vi "Send YIELD.vi"(8 "error in (no error)":errorcluster, 9 "Yield request":T1={"Invocation Request ID"=0, "Arguments"=[], "ArgumentsKw"="{}", "Options"="{}"}, 11 "WAMP Client in":refnum<class "WAMP Client.lvclass">) -> (0 "error out":errorcluster, 3 "WAMP Client out":refnum<class "WAMP Client.lvclass">)   [LabVIEW 2020, in "wamplv.lvlib" / "WAMP Client.lvclass"]
uses:
  WAMP Client.lvclass
  TypeDef/YIELD request data.ctl
  TypeDef/WAMP Message Codes.ctl
  WAMP Client.lvclass/WAMP Client.ctl
  <vilib>/JDP Science/JSONtext/JSONtext.lvlib
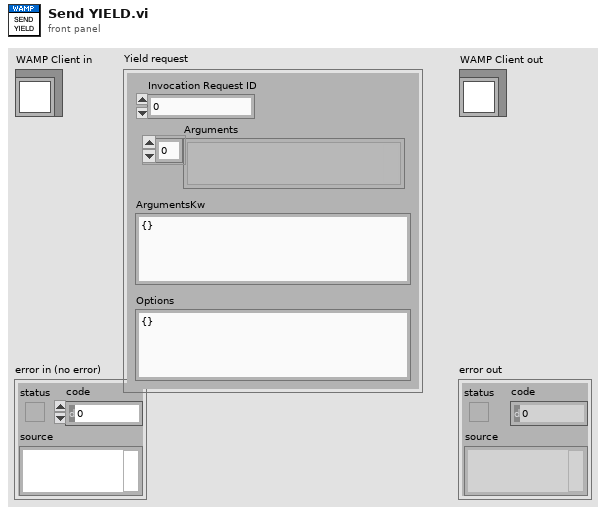
[diagram p1: front panel]
types:
  T1 = typedef "wamplv.lvlib/WAMP Client.lvclass/YIELD request data.ctl" = cluster{"Invocation Request ID":u64, "Arguments":variant[], "ArgumentsKw":string, "Options":string}
  T2 = typedef "wamplv.lvlib/WAMP Client.lvclass/WAMP Message Codes.ctl" = u16
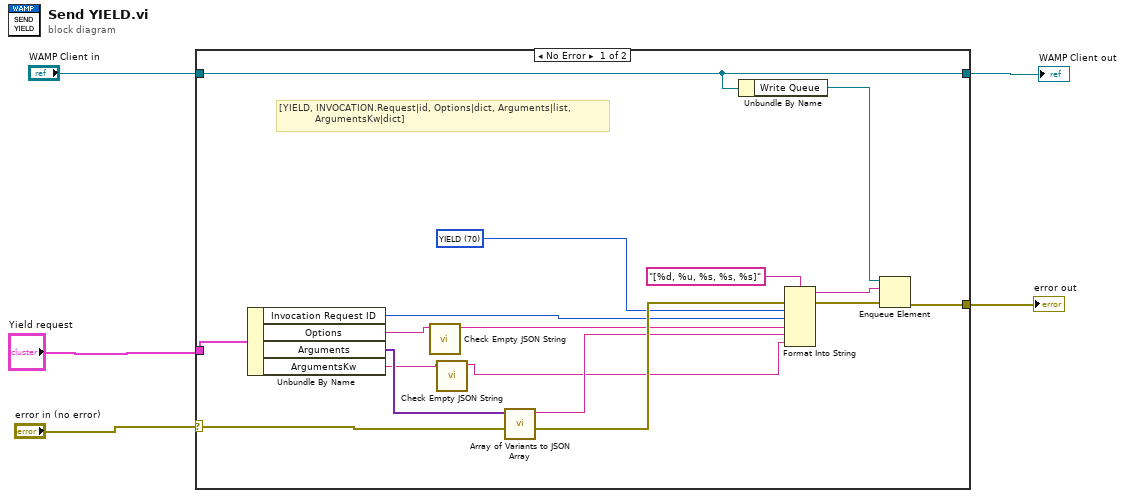
[diagram p0: block diagram]
diagram:
  n1 = case shown="No Error" "error in (no error)" {
    selector: "error in (no error)" -> [w17 w24]
    tunnel: [w22 w24] -> w4
    tunnel: [w15 w23] -> w2
    tunnel: "WAMP Client in" -> [w15 w23]
    tunnel: "Yield request" -> [w13 _]
    frame No Error {
      w14 = T2 70 items=["HELLO"=1, "WELCOME"=2, "ABORT"=3, "GOODBYE"=6, "ERROR"=8, "PUBLISH"=16, "PUBLISHED"=17, "SUBSCRIBE"=32, "SUBSCRIBED"=33, "UNSUBSCRIBE"=34, "UNSUBSCRIBED"=35, "EVENT"=36, "CALL"=48, "RESULT"=59, "REGISTER"=64, "REGISTERED"=65, "UNREGISTER"=66, "UNREGISTERED"=67, "INVOCATION"=68, "YIELD"=70] ("Message Codes")
      # "[YIELD, INVOCATION.Request|id, Options|dict, Arguments|list,\n            ArgumentsKw|dict]"
      n2 = Unbundle By Name(w13) -> ("Invocation Request ID"=w12:u64, "Options"=w7:string, "Arguments"=w11:variant[], "ArgumentsKw"=w9:string)
      n3 = call "Check Empty JSON String.vi"("JSON"=w7) -> ("JSON"=w6:string)  [unwired: 10 in]
      n4 = call "Check Empty JSON String.vi"("JSON"=w9) -> ("JSON"=w8:string)  [unwired: 10 in]
      n5 = call <vilib>:"Array of Variants to JSON Array.vi"("error in (no error)"=w17, "Array of Variants"=w11) -> ("error out"=w16:errorcluster, "<JSON>"=w10:string)  [unwired: 8 in]
      n6 = Unbundle By Name(w15) -> ("Write Queue"=w18:refnum<queue>)
      n7 = Format Into String(format string="[%d, %u, %s, %s, %s]" ("element"), error in=w16, w14, w12, w6, w10, w8) -> (resulting string=w20:string, error out=w19:errorcluster)  [unwired: 1 in]
      n8 = Enqueue Element(queue=w18, element=w20, error in (no error)=w19) -> (error out=w22:errorcluster)  [unwired: 1 in, 2 out]
    }
    frame Error {
    }
  }
  "error out" <- w4
  "WAMP Client out" <- w2
